vi "CU_TrainMahalanobis.vi"(6 "DataTypes":T1, 8 "error in (no error)":errorcluster, 10 "Indices":i8[](array[numeric]), 11 "ClassifierClass in":refnum<class "ClassifierClass.lvclass">) -> (0 "error out":errorcluster, 1 "Mean vectors":dbl[][](array[numeric]), 2 "Covariance matricies":dbl[][][](array[numeric]), 3 "ClassifierClass out":refnum<class "ClassifierClass.lvclass">)   [LabVIEW 2016, in "Classifier.lvlib" / "ClassifierClass.lvclass"]
uses:
  ClassifierClass.lvclass
  CU_DataTypes.ctl
  ClassifierClass.lvclass/ClassifierClass.ctl
  <vilib>/Analysis/baseanly.llb/Real Inverse Matrix.vi
  <vilib>/gmath/NI_Gmath.lvlib
  <vilib>/Analysis/NI_AALBase.lvlib
  Classifier.lvlib
panel:
  out "Sizes":i32[](array[numeric])
  # "This VI is a part of BCI Design library, http://www.ru-bci.org \nCopyright © 2020, Sotnikov Peter, All rights reserved. License: GNU GPLv3"
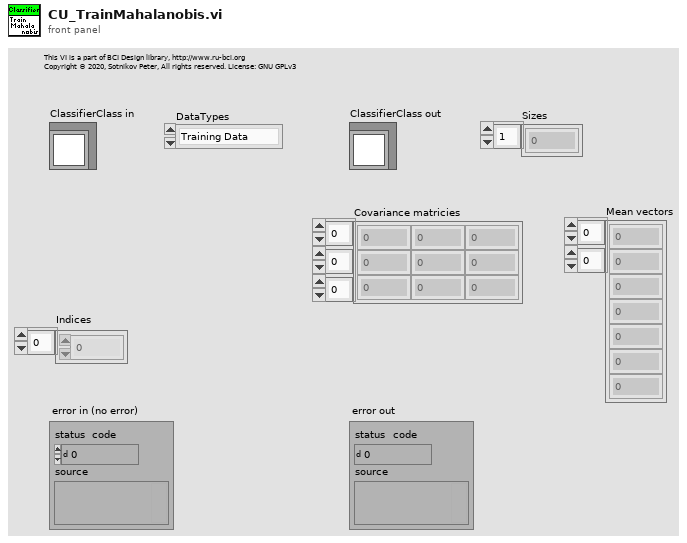
[diagram p1: front panel]
types:
  T1 = typedef "Classifier.lvlib/CU_DataTypes.ctl" = enum16{"Training Data", "Test Data", "Training Data (cross-check)", "Test Data (cross-check)"}
  T2 = typedef "XML_EEG_Features.lvlib/XML_FF_Trial.ctl" = cluster{"ClassLabel":string, "FeatureVector":dbl[]}
  T3 = typedef "NI_Matrix.lvlib/RealMatrix.ctl" = dbl[][]
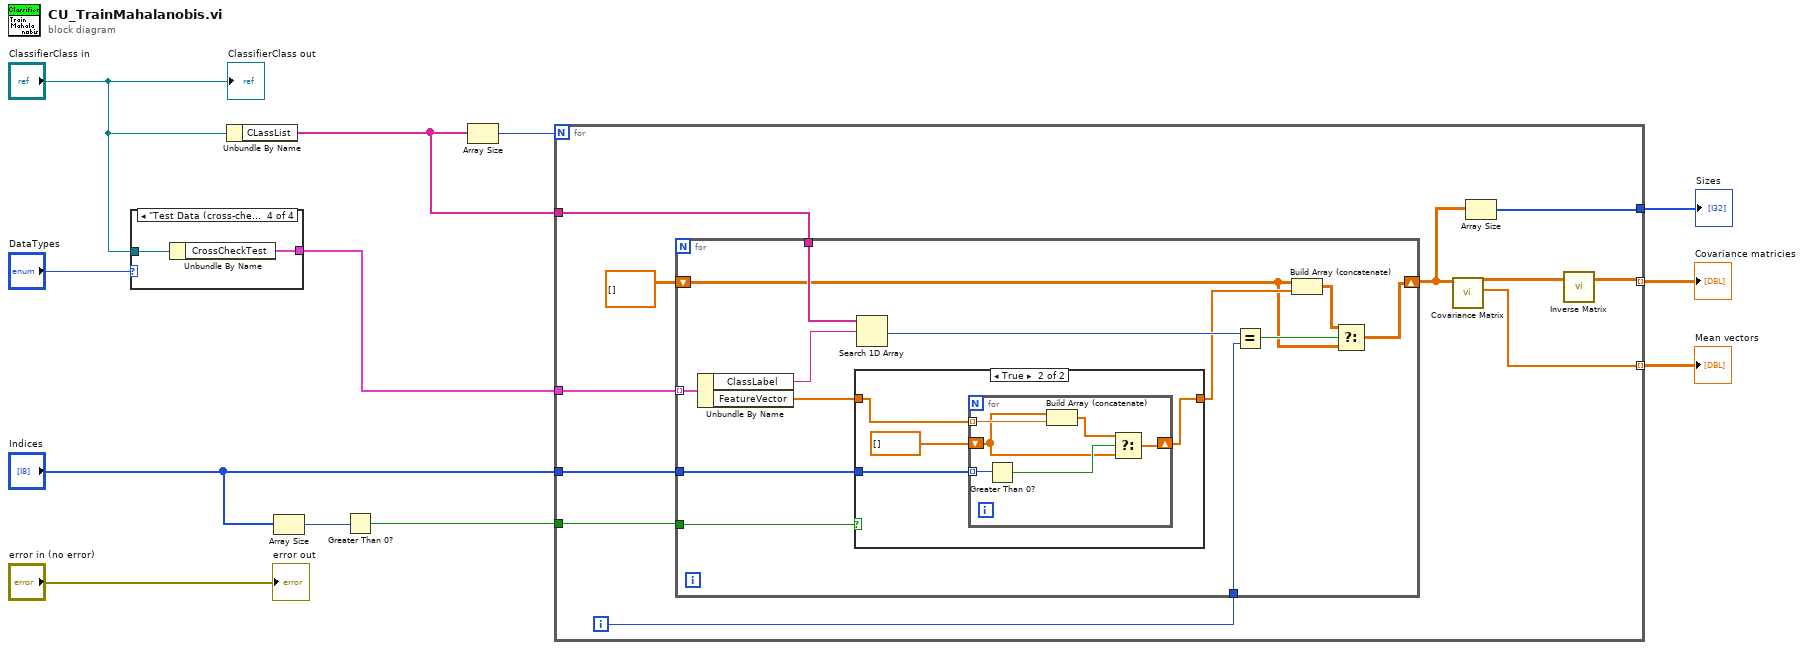
[diagram p0: block diagram]
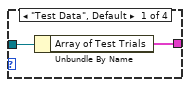
[diagram p2: hidden frame]
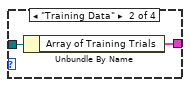
[diagram p3: hidden frame]
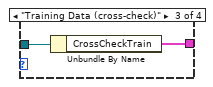
[diagram p4: hidden frame]
diagram:
  n1 = case shown="\"Test Data (cross-check)\"" "DataTypes" {
    tunnel: "ClassifierClass in" -> [w14 w16 w18 w20]
    tunnel: [w13 w15 w17 w19] -> w1
    frame "Test Data", Default {
      n2 = Unbundle By Name(w14) -> ("Array of Test Trials"=w13:T2[])
    }
    frame "Training Data" {
      n3 = Unbundle By Name(w16) -> ("Array of Training Trials"=w15:T2[])
    }
    frame "Training Data (cross-check)" {
      n4 = Unbundle By Name(w18) -> ("CrossCheckTrain"=w17:T2[])
    }
    frame "Test Data (cross-check)" {
      n5 = Unbundle By Name(w20) -> ("CrossCheckTest"=w19:T2[])
    }
  }
  n6 = Unbundle By Name("ClassifierClass in") -> ("CLassList"=w8:string[])
  n7 = Array Size(array="Indices") -> (size(s)=w12:i32)
  n8 = Greater Than 0?(x=w12) -> (x > 0?=w11:bool)
  n9 = Array Size(array=w8) -> (size(s)=w9:i32)
  n10 = for {
    N: w9 -> [_]
    tunnel: w11 -> [w31]
    tunnel: "Indices" -> [w30]
    tunnel: w1 -> [w29]
    tunnel: w8 -> [w28]
    tunnel: [w21] -> w5 mode=indexing
    tunnel: [w25] -> w4 mode=indexing
    tunnel: [w23] -> w6
    i -> [w27]
    n11 = for {
      tunnel: w29 -> [w44] mode=indexing
      tunnel: w30 -> [w42]
      tunnel: w31 -> [w41]
      tunnel: w28 -> [w40]
      tunnel: w27 -> [w37]
      shift-right: [w32] -> w24
      shift-left: dbl[][] [] -> [w33]
      n12 = Unbundle By Name(w44) -> ("ClassLabel"=w39:string, "FeatureVector"=w43:dbl[])
      n13 = case shown="True" w41 {
        tunnel: w43 -> [w45 w49]
        tunnel: [w45 w46] -> w35
        tunnel: w42 -> [_ w48]
        frame False {
        }
        frame True {
          n14 = for {
            tunnel: w49 -> [w52] mode=indexing
            tunnel: w48 -> [w55] mode=indexing
            shift-right: [w54] -> w46
            shift-left: dbl[] [] -> [w50]
            n15 = Greater Than 0?(x=w55) -> (x > 0?=w53:bool)
            n16 = Build Array (concatenate)(w50, w52) -> (w51:dbl[])
            n17 = Select(t=w51, s=w53, f=w50) -> (s? t:f=w54:dbl[])
          }
        }
      }
      n18 = Search 1D Array(1D array=w40, element=w39) -> (index of element=w38:i32)  [unwired: 1 in]
      n19 = Equal?(x=w38, y=w37) -> (x = y?=w36:bool)
      n20 = Build Array (concatenate)(w33, w35) -> (w34:dbl[][])
      n21 = Select(t=w34, s=w36, f=w33) -> (s? t:f=w32:dbl[][])
    }
    n22 = call <vilib>:"Covariance Matrix.vi"("X"=w24) -> ("mean vector"=w25:dbl[], "covariance matrix V"=w22:T3)  [unwired: 9 in]
    n23 = Array Size(array=w24) -> (size(s)=w23:i32[])
    n24 = call-poly <vilib>:"Inverse Matrix.vi"("Input Matrix"=w22) -> ("Inverse Matrix"=w21:T3)  [unwired: 1 in, 1 out]
  }
  "Sizes" <- w6
  "Covariance matricies" <- w5
  "Mean vectors" <- w4
  "error out" <- "error in (no error)"
  "ClassifierClass out" <- "ClassifierClass in"
